vi "Dresser DXD Error Message.vi"(0 "VISA session":refnum<visa-resource-name>, 11 "Error In (no error)":errorcluster) -> (3 "Status":bool, 4 "dup VISA session":refnum<visa-resource-name>, 8 "Error Code (0)":i32, 10 "Error Message (empty)":string, 15 "Error Out":errorcluster)   [LabVIEW 2015]
doc: "This VI contains all the Dresser DXD Series pressure transducer specific error codes and descriptions. Use this VI after executing several instrument driver VIs to recognize and display any errors that may have occurred.\n\nCode from User Defined User Defined\nTransducer Code Descriptions\n-----------------------------------------------------------------------------------------------------------------------------------------------\nErr01 5001 Err01 - ADC no response within 300 ms.\nErr02 5002 Err02 - EEPROM write error.\nErr03 5003 Err03 - Incorrect numerical format for command.\nErr04 5004 Err04 - Calculated output over range.\nErr05 5005 Err05 - ADC over range. Either channel 1 or 2.\nErr06 5006 Err06 - Bad pressure type value.\nErr07 5007 Err07 - Illegal scale factor. Either channel 1 or 2.\nErr08 5008 Err08 - ADC reference voltage unstable or not present.\n\nWritten by:\nBLOOMY CONTROLS, INC\nWINDSOR, CT 06095, USA\n860-298-9925\nwww.bloomy.com\nV2.0.0\nMay, 2002"
panel:
  in  "Type of Dialog (1: OK Msg)":i32(ring)=1 items=["No Dialog", "OK Message", "Continue or Stop Message"]
  in  "User-Defined Descriptions":string[](array[string])=["Err01 - ADC no response within 300 ms.", "Err02 - EEPROM write error.", "Err03 - Incorrect numerical format for command.", "Err04 - Calculated output over range.", "Err05 - ADC over range.  Either channel 1 or 2.", "Err06 - Bad pressure type value.", "Err07 - Illegal scale factor.  Either channel 1 or 2.", "Err08 - ADC reference voltage unstable or not present."]
  in  "User-Defined Codes":i32[](array[numeric])=[5001, 5002, 5003, 5004, 5005, 5006, 5007, 5008]
  # "For instructions on the use of this VI, press Ctrl+H to display the help window and move the mouse over the icon, controls, and indicators"
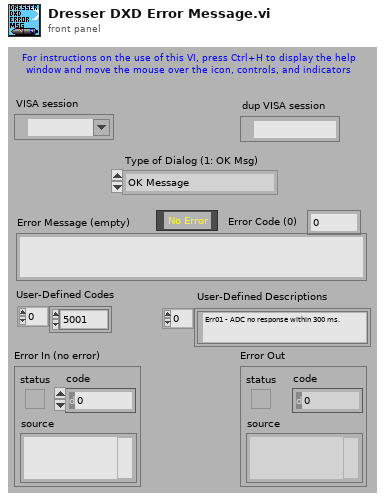
[diagram p1: front panel]
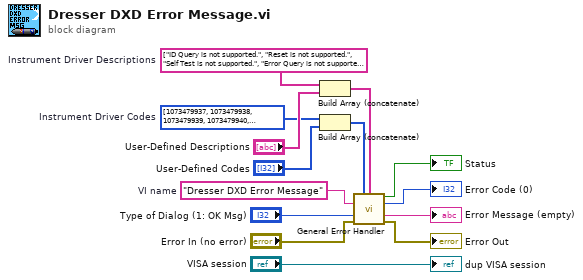
[diagram p0: block diagram]
diagram:
  w3 = i32[] [1073479937, 1073479938, 1073479939, 1073479940, 1073479941, -1074003951, -1074001917, -1074001665, 0]  # Instrument Driver Codes
  w6 = string[] ["ID Query is not supported.", "Reset is not supported.", "Self Test is not supported.", "Error Query is not supported.", "Revision Query is not supported.", "Invalid Response to Instrument ID Query.", "Error Interpreting Instrument Response.", "Instrument Specific Error Occurred.", ""]  # Instrument Driver Descriptions
  w11 = "Dresser DXD Error Message"  # VI name
  n1 = Build Array (concatenate)(w6, "User-Defined Descriptions") -> (w2:string[])
  n2 = Build Array (concatenate)(w3, "User-Defined Codes") -> (w1:i32[])
  n3 = call <vilib>:"General Error Handler.vi"("[user-defined codes]"=w1, "[user-defined descriptions]"=w2, "[error source] (\" \")"=w11, "type of dialog (OK msg:1)"="Type of Dialog (1: OK Msg)", "error in (no error)"="Error In (no error)") -> ("error?"=→"Status":bool, "code out"=→"Error Code (0)":i32, "message"=→"Error Message (empty)":string, "error out"=→"Error Out":errorcluster)  [unwired: 6 in, 1 out]
  "dup VISA session" <- "VISA session"
